vi "FestoCPX.Valve(2out1in).vi"(4 "negate input (F)":bool, 6 "Timeout [ms] (5000)":u32=5000, 8 "error in (no error)":errorcluster, 9 "Position":T3, 10 "Outputs":T2[](array[typedef]), 11 "Input":T1) -> (0 "error out":errorcluster, 2 "Aborted?":bool, 3 "Timeout?":bool)   [LabVIEW 2016]
uses:
  Station/Station.ValvePosition.ctl
  FestoCPX.DO.Signal.ctl
  FestoCPX.DI.Signal.ctl
  FestoCPX.DI.Data.State.Get.vi
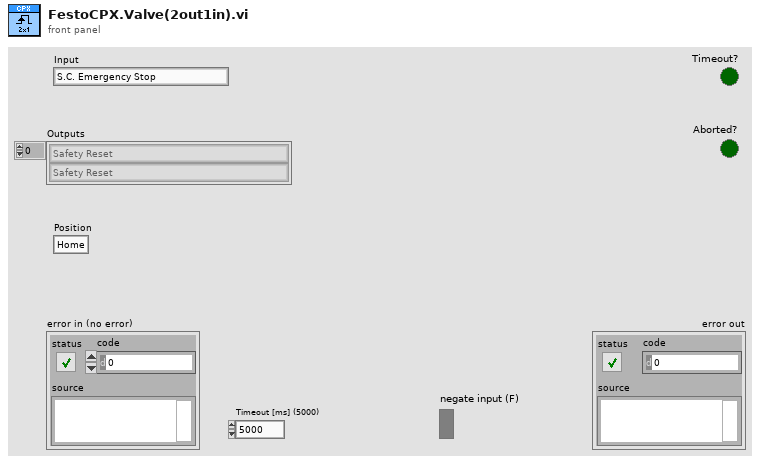
[diagram p1: front panel]
types:
  T1 = typedef "FestoCPX.DI.Signal.ctl" = enum16{"S.C. Emergency Stop", "S.C. Side Door Close", "S.C. Front Door Close", "S.C. Front Door Secured", "Button Start", "Button Stop", "Button Control", "Product Move Home", "Product Move Work", "Table Position", "Table Lock", "Product Lift A Home", "Product Lift B Home", "Product Arm OK", "Product Arm NOK", "Product Arm Work", "Revolver ID 1", "Revolver ID 2", "Revolver ID 3", "Revolver ID 4", "Revolver ID 5", "Air Pressure Inside", "Air Pressure Inlet", "Product Slot 1 A Present", "Product Slot 1 B Present", "Product Slot 2 A Present", "Product Slot 2 B Present", "Product Slot 3 A Present", "Product Slot 3 B Present", "Product Slot 4 A Present", "Product Slot 4 B Present", "Product Final A Present", "Product Final B Present", "Product Output A Present", "Product Output B Present", "Product Container OK Present", "Product Container NOK Present", "Fork ID 1", "Fork ID 2"}
  T2 = typedef "FestoCPX.DO.Signal.ctl" = enum16{"Safety Reset", "Air Main Valve", "Door Lock", "Button LED Start", "Button LED Stop", "Button LED Control", "Traffic LED Red", "Traffic LED Orange", "Traffic LED Green", "Horn", "Laser Interlock", "Laser Trigger", "Laser Fume Extractor", "Product Suction Gripper Slot 1 A", "Product Suction Gripper Slot 1 B", "Product Suction Gripper Slot 2 A", "Product Suction Gripper Slot 2 B", "Product Suction Gripper Slot 3 A", "Product Suction Gripper Slot 3 B", "Product Suction Gripper Slot 4 A", "Product Suction Gripper Slot 4 B", "Product Suction Gripper Final A", "Product Suction Gripper Final B", "Lamp", "Q1 Product Move Work", "Q1 Product Move Home", "Q2 Table Turn Work", "Q2 Table Turn Home", "Q3 Product Lift A", "Q3 Product Lift B", "Q4 Product Arm OK", "Q4 Product Arm NOK", "Q5 Product Arm Work", "Q6 Product BlowOut A", "Q6 Product BlowOut B"}
  T3 = typedef "Station.ValvePosition.ctl" = enum16{"Home", "Work"}
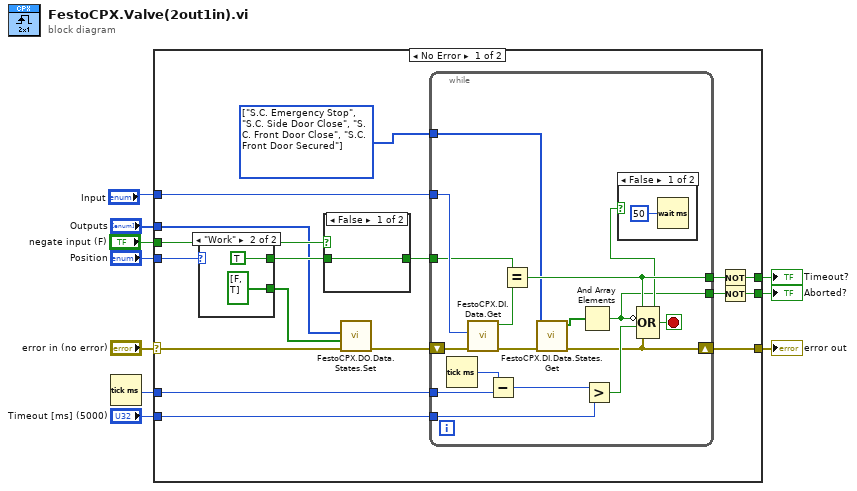
[diagram p0: block diagram]
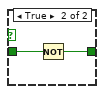
[diagram p2: hidden frame]
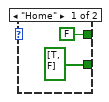
[diagram p4: hidden frame]
diagram:
  n1 = Tick Count (ms)() -> (millisecond timer value=w6:u32)
  n2 = case shown="No Error" "error in (no error)" {
    selector: "error in (no error)" -> [w17 w52]
    tunnel: "Position" -> [w25 _]
    tunnel: [w21 w52] -> w9
    tunnel: [w23 _] -> w8
    tunnel: w6 -> [w27 _]
    tunnel: "Timeout [ms] (5000)" -> [w26 _]
    tunnel: "Input" -> [w24 _]
    tunnel: "Outputs" -> [w14 _]
    tunnel: "negate input (F)" -> [w19 _]
    tunnel: [w11 _] -> w1
    frame No Error {
      w13 = T1[] [enum."S.C. Emergency Stop", enum."S.C. Side Door Close", enum."S.C. Front Door Close", enum."S.C. Front Door Secured"] items=["S.C. Emergency Stop", "S.C. Side Door Close", "S.C. Front Door Close", "S.C. Front Door Secured", "Button Start", "Button Stop", "Button Control", "Product Move Home", "Product Move Work", "Table Position", "Table Lock", "Product Lift A Home", "Product Lift B Home", "Product Arm OK", "Product Arm NOK", "Product Arm Work", "Revolver ID 1", "Revolver ID 2", "Revolver ID 3", "Revolver ID 4", "Revolver ID 5", "Air Pressure Inside", "Air Pressure Inlet", "Product Slot 1 A Present", "Product Slot 1 B Present", "Product Slot 2 A Present", "Product Slot 2 B Present", "Product Slot 3 A Present", "Product Slot 3 B Present", "Product Slot 4 A Present", "Product Slot 4 B Present", "Product Final A Present", "Product Final B Present", "Product Output A Present", "Product Output B Present", "Product Container OK Present", "Product Container NOK Present", "Fork ID 1", "Fork ID 2"] ("CPX.DI")
      n3 = case shown="\"Work\"" w25 {
        tunnel: [bool[] [TRUE, FALSE] bool[] [FALSE, TRUE]] -> w15
        tunnel: [FALSE TRUE] -> w20
        frame "Home" {
        }
        frame "Work" {
        }
      }
      n4 = case shown="False" w19 {
        tunnel: w20 -> [w28 w30]
        tunnel: [w28 w29] -> w18
        frame False {
        }
        frame True {
          n5 = Not(x=w30) -> (.not. x?=w29:bool)
        }
      }
      n6 = call "FestoCPX.DO.Data.States.Set.vi"("error in (no error)"=w17, "State"=w15, "CPX.DO"=w14) -> ("error out"=w16:errorcluster)  [unwired: 8 in]
      n7 = while {
        shift-right: [w34] -> w21
        shift-left: w16 -> [w46]
        tunnel: w24 -> [w45]
        tunnel: [w38] -> w22
        tunnel: w27 -> [w43]
        tunnel: w26 -> [w41]
        tunnel: w18 -> [w39]
        tunnel: w13 -> [w35]
        tunnel: [w33] -> w12
        stop <- w37 stop-if-true
        n8 = Tick Count (ms)() -> (millisecond timer value=w44:u32)
        n9 = call-poly "FestoCPX.DI.Data.Get.vi"("error in (no error)"=w46, "CPX.DI"=w45) -> ("error out"=w36:errorcluster, "State"=w31:bool)  [unwired: 5 in, 3 out]
        n10 = Subtract(x=w44, y=w43) -> (x-y=w42:u32)
        n11 = Equal?(x=w39, y=w31) -> (x = y?=w38:bool)
        n12 = call "FestoCPX.DI.Data.States.Get.vi"("error in (no error)"=w36, "CPX.DI"=w35) -> ("error out"=w34:errorcluster, "State"=w32:bool[])  [unwired: 5 in, 3 out]
        n13 = And Array Elements(Boolean array=w32) -> (logical AND=w33:bool)
        n14 = Greater?(x=w42, y=w41) -> (0:w40:bool)
        n15 = Compound Arithmetic op=OR(w38, invert w33, w40, w34) -> (w37:bool)
        n16 = case shown="False" w37 {
          frame False {
            n17 = Wait (ms)(milliseconds to wait=u32 50) -> ()  [unwired: 1 out]
          }
          frame True {
          }
        }
      }
      n18 = Not(x=w22) -> (.not. x?=w23:bool)
      n19 = Not(x=w12) -> (.not. x?=w11:bool)
    }
    frame Error {
    }
  }
  "error out" <- w9
  "Timeout?" <- w8
  "Aborted?" <- w1
